vi "VI Tester JUnitXML Example.vi"() -> ()   [LabVIEW 2013]
uses:
  TextTestRunner.JUnitXML/TextTestRunner.JUnitXML.lvclass
  <vilib>/Utility/sysdir.llb/System Directory Type.ctl
  <userlib>/_OpenG.lib/file/file.llb/Append Path to Root if Relative - Scalar__ogtk.vi
  <vilib>/addons/_JKI Toolkits/VI Tester/VI Tester API.llb/Run Tests (Path).vi
  <vilib>/addons/_JKI Toolkits/VI Tester/VI Tester API.llb/VI Tester API.lvlib
panel:
  out "JUnit XML report":string
  in  "Test Path":path=path "examples/JKI/VI Tester/Queue TestCase/Queue TestCase.lvclass"
  out "error out":errorcluster
  out "test details":string
  out "successful?":bool
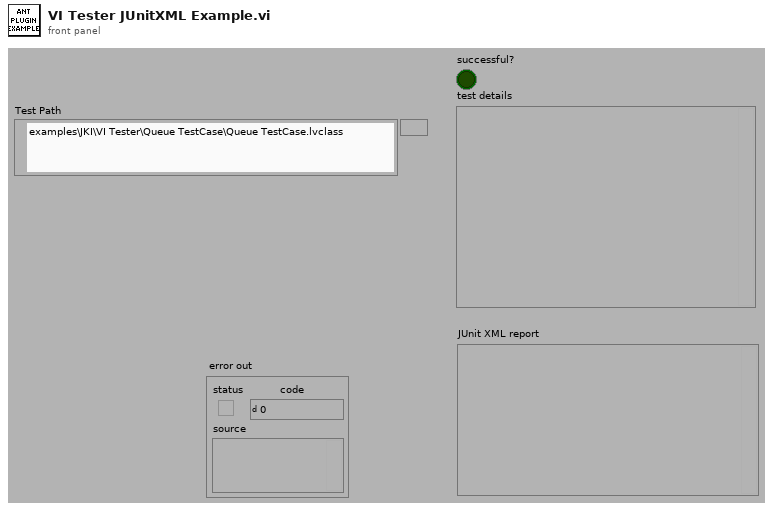
[diagram p1: front panel]
types:
  T1 = typedef "System Directory Type.ctl" = i32
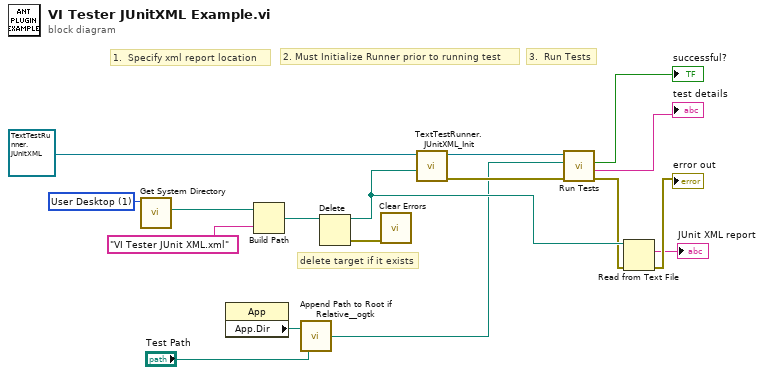
[diagram p0: block diagram]
diagram:
  w16 = T1 1 items=["User Home", "User Desktop", "User Documents", "User Application Data", "User Preferences", "User Temporary", "Public Documents", "Public Application Data", "Public Preferences", "System Core Libraries", "System Installed Libraries", "Application Files", "Boot Volume Root"] ("system directory type")
  # "3.  Run Tests"
  # "delete target if it exists"
  # "2. Must Initialize Runner prior to running test"
  # "1.  Specify xml report location"
  n1 = call <vilib>:"Get System Directory.vi"("system directory type"=w16) -> ("system directory"=w15:path)  [unwired: 10 in]
  n2 = property class="App"() -> ("App.Dir"=w2:path)  [unwired: 2 in, 2 out]
  n3 = Build Path(base path=w15, name or relative path="VI Tester JUnit XML.xml") -> (appended path=w9:path)
  n4 = call-poly <userlib>:"Append Path to Root if Relative__ogtk.vi"("Absolute or Relative Path"="Test Path", "Root Path"=w2) -> ("Absolute or Appended Path"=w3:path)
  n5 = Delete(path (use dialog)=w9) -> (deleted path=w7:path, error out=w8:errorcluster)  [unwired: 4 in, 1 out]
  n6 = call <vilib>:"Clear Errors.vi"("error in (no error)"=w8) -> ()  [unwired: 6 in, 1 out]
  n7 = call "TextTestRunner.JUnitXML_Init.vi"("Report Path"=w7, "TextTestRunner in"=refnum<class "TextTestRunner.JUnitXML.lvclass"> refnum ("TextTestRunner.Ant.lvclass")) -> ("error out"=w10:errorcluster, "TextTestRunner out"=w11:refnum<class "TextTestRunner.JUnitXML.lvclass">)  [unwired: 8 in]
  n8 = call-poly <vilib>:"Run Tests.vi"("TextTestRunner in"=w11, "error in (no error)"=w10, "Test Path"=w3) -> ("error out"=w6:errorcluster, "test details"=→"test details":string, "successful?"=→"successful?":bool)  [unwired: 6 in]
  n9 = Read from Text File(file (use dialog)=w7, error in=w6) -> (text=→"JUnit XML report":string, error out=→"error out":errorcluster)  [unwired: 2 in, 2 out]
